vi "Power Accuracy Build Key Array for Config.vi"(8 "error in (no error)":errorcluster, 9 "Power Accuracy Test Parameters":T2={"Stimulus"={"Power Start"=38, "Power Stop"=46, "Frequency Type"=enum."Band Edges", "Frequency Points"=[], "TX 1 Frequency (MHz)"={"Min"=0.0, "Max"=0.0}, "TX 2 Frequency (MHz)"={"Min"=0.0, "Max"=0.0}, "RX Frequency (MHz)"={"Min"=0.0, "Max"=0.0}, "Pad Model Number"="", "Pad Serial Number"="", "Pad Values"=[]}, "Measurement"={"DUT Port"=enum."Port 1", "Direction"=0}, "Display"={"Power"={"Min"=0, "Max"=0}, "Tolerance"={"Min"=0.0, "Max"=0.0}}, "Limit"={"Tolerance"=0.35}, "Calibration"={"Calibrated?"=FALSE}} {"Measurement"."Direction" items=["Reverse", "Forward", "Auxiliary"]}, 10 "Key Array In":T10, 11 "Connection Refnum":T1) -> (0 "error out":errorcluster, 2 "Key Array Out":T10, 3 "Connection Refnum":T1)   [LabVIEW 2011]
uses:
  Addons/internet/utils/keyedarr.llb/Keyed Array.ctl
  TypeDefs/Power Accuracy Test Parameters.ctl
  TypeDefs/Power Accuracy Stimulus Parameters.ctl
  TypeDefs/Power Accuracy Measurement Parameters.ctl
  SI.LIB/PIM.LIB/HW IO/DUTport.ctl
  SI.LIB/PIM.LIB/HW IO/MeasMode.ctl
  TypeDefs/Power Accuracy Display Parameters.ctl
  TypeDefs/Power Accuracy Limit Parameters.ctl
  TypeDefs/Power Accuracy Calibration State.ctl
  SI.LIB/ODBC/SQL Controls/Connection Refnum.ctl
  Addons/internet/utils/strutil.llb/Case Matching.ctl
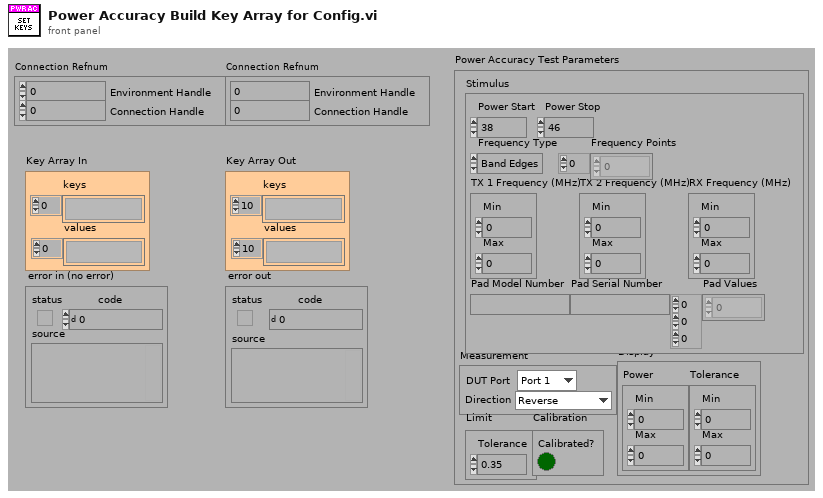
[diagram p1: front panel]
types:
  T1 = typedef "Connection Refnum.ctl" = cluster{"Environment Handle":i32, "Connection Handle":i32}
  T2 = typedef "Power Accuracy Test Parameters.ctl" = cluster{"Stimulus":T3, "Measurement":T4, "Display":T7, "Limit":T8, "Calibration":T9}
  T3 = typedef "Power Accuracy Stimulus Parameters.ctl" = cluster{"Power Start":i32, "Power Stop":i32, "Frequency Type":enum16{"Band Edges", "Custom"}, "Frequency Points":dbl[], "TX 1 Frequency (MHz)":cluster{"Min":dbl, "Max":dbl}, "TX 2 Frequency (MHz)":cluster{"Min":dbl, "Max":dbl}, "RX Frequency (MHz)":cluster{"Min":dbl, "Max":dbl}, "Pad Model Number":string, "Pad Serial Number":string, "Pad Values":dbl[][][]}
  T4 = typedef "Power Accuracy Measurement Parameters.ctl" = cluster{"DUT Port":T5, "Direction":T6}
  T5 = typedef "DUTport.ctl" = enum16{"Port 1", "Port 2"}
  T6 = typedef "MeasMode.ctl" = u16
  T7 = typedef "Power Accuracy Display Parameters.ctl" = cluster{"Power":cluster{"Min":i32, "Max":i32}, "Tolerance":cluster{"Min":dbl, "Max":dbl}}
  T8 = typedef "Power Accuracy Limit Parameters.ctl" = cluster{"Tolerance":dbl}
  T9 = typedef "Power Accuracy Calibration State.ctl" = cluster{"Calibrated?":bool}
  T10 = typedef "Keyed Array.ctl" = cluster{"keys":string[], "values":string[]}
  T11 = typedef "Case Matching.ctl" = enum16{"a != A", "a == A", "system"}
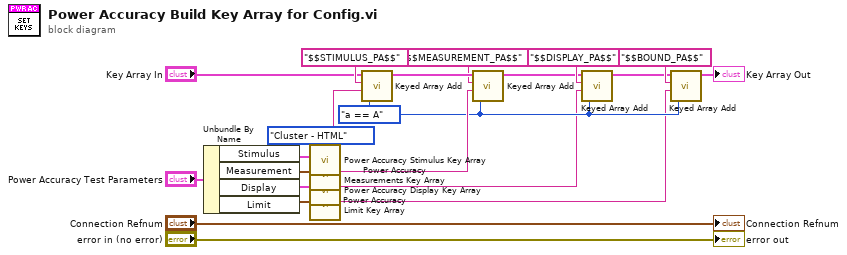
[diagram p0: block diagram]
diagram:
  w11 = Case_Matching."a == A" ("case matching (sensitive)")
  w10 = enum16{"Cluster - HTML", "HTML - Cluster"}."Cluster - HTML" ("Conversion")
  n1 = Unbundle By Name("Power Accuracy Test Parameters") -> ("Stimulus"=w13:T3, "Measurement"=w12:T4, "Display"=w1:T7, "Limit"=w2:T8)
  n2 = call "Power Accuracy Stimulus Key Array.vi"("Conversion"=w10, "Stimulus Cluster In"=w13) -> ("Stimulus HTML Out"=w18:string)  [unwired: 5 in, 1 out]
  n3 = call "Power Accuracy Measurements Key Array.vi"("Conversion"=w10, "Measurements Cluster In"=w12) -> ("Measurements HTML Out"=w16:string)  [unwired: 5 in, 1 out]
  n4 = call "Power Accuracy Display Key Array.vi"("Conversion"=w10, "Display Cluster In"=w1) -> ("Display HTML Out"=w4:string)  [unwired: 5 in, 1 out]
  n5 = call "Power Accuracy Limit Key Array.vi"("Conversion"=w10, "Limits Cluster In"=w2) -> ("Limits HTML Out"=w3:string)  [unwired: 5 in, 1 out]
  n6 = call "Keyed Array Add.vi"("case matching (sensitive)"=w11, "value"=w18, "key"="$$STIMULUS_PA$$", "array in"="Key Array In") -> ("array out"=w20:T10)  [unwired: 3 out]
  n7 = call "Keyed Array Add.vi"("case matching (sensitive)"=w11, "value"=w16, "key"="$$MEASUREMENT_PA$$", "array in"=w20) -> ("array out"=w5:T10)  [unwired: 3 out]
  n8 = call "Keyed Array Add.vi"("case matching (sensitive)"=w11, "value"=w4, "key"="$$DISPLAY_PA$$", "array in"=w5) -> ("array out"=w6:T10)  [unwired: 3 out]
  n9 = call "Keyed Array Add.vi"("case matching (sensitive)"=w11, "value"=w3, "key"="$$BOUND_PA$$", "array in"=w6) -> ("array out"=→"Key Array Out":T10)  [unwired: 3 out]
  "error out" <- "error in (no error)"
  "Connection Refnum" <- "Connection Refnum"
